vi "deleteFileCategory.vi"(1 "VarableID":T1) -> ()   [LabVIEW 2010]
uses:
  VarableID.ctl
  AmmeterGlobalCostants.vi
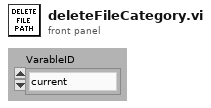
[diagram p1: front panel]
types:
  T1 = typedef "VarableID.ctl" = enum16{"current", "power", "PF", "voltage"}
  T2 = typedef "VarableStruct.ctl" = cluster{"Name":string, "StorageRefnum":refnum<file>, "Command":string, "IsDetecting":bool, "VarableID":T1}
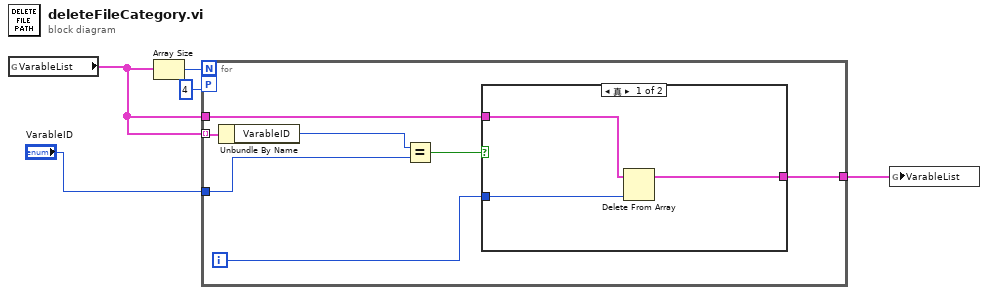
[diagram p0: block diagram]
diagram:
  n1 = global read "AmmeterGlobalCostants.vi" "VarableList"() -> (w4:T2[])
  n2 = Array Size(array=w4) -> (size(s)=w5:i32)
  n3 = for "For循环" {
    N: w5 -> [_]
    tunnel: "VarableID" -> [w7]
    tunnel: w4 -> [w8] mode=indexing
    tunnel: w4 -> [w11]
    tunnel: [w9] -> w2
    workers-P: 4 -> [_]
    i -> [w10]
    n4 = Unbundle By Name(w8) -> ("VarableID"=w6:T1)
    n5 = Equal?(x=w6, y=w7) -> (x = y?=w12:bool)
    n6 = case shown="真" w12 {
      tunnel: w11 -> [w15 w16]
      tunnel: w10 -> [w14 _]
      tunnel: [w13 w16] -> w9
      frame True {
        n7 = Delete From Array(array=w15, index=w14) -> (array with subset deleted=w13:T2[])  [unwired: 1 in, 1 out]
      }
      frame False {
      }
    }
  }
  n8 = global write "AmmeterGlobalCostants.vi" "VarableList"(w2) -> ()
